vi "Combination Test.vi"() -> ()   [LabVIEW 2024]
uses:
  Log Record.ctl
  Logger/Internal Log Levels.ctl
  Filters/Match Behavior.ctl
  Filters/Aggregation Method.ctl
  5a9499bb-b307-4a4d-bae3-2140953a7cf6.vi
  5a9499bb-b307-4a4d-bae3-2140953a7cf6.vi/a153a250-4fb8-4a99-bb5b-6ccb57f1f631.vi
  5a9499bb-b307-4a4d-bae3-2140953a7cf6.vi/a153a250-4fb8-4a99-bb5b-6ccb57f1f631.vi/28727e37-b0d9-407c-a479-ab0b7779cd69.vi
  Filters/Regex/Regex.lvclass
  Handlers/File Handler/File Handler.lvclass
  Filters/Combination/Combination.lvclass
  Filters/Regex/New (Element).vi
  Registry/Log.vi
  Registry/Registry.lvlib
  Logger/Logger.lvclass
  Logging.lvlib
  Filters/Scopes/Scope/Scope.lvclass
panel:
  out "error out":errorcluster
  out "failures":T3(array[cluster]) {"Log Record"."timestamp" format="%<%x %.3X>T"}
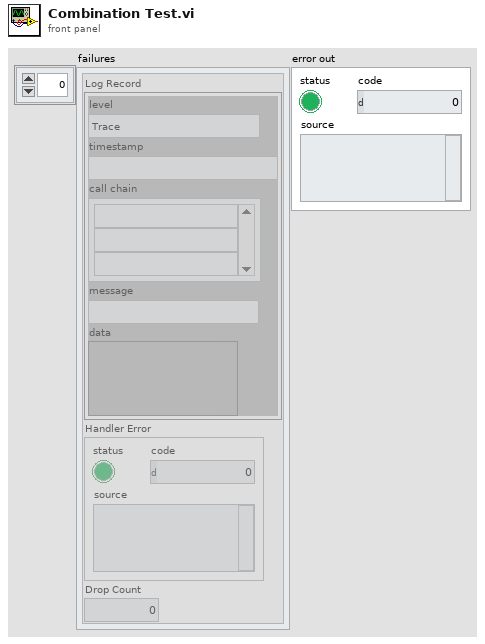
[diagram p1: front panel]
types:
  T1 = typedef "Logging.lvlib/Log Record.ctl" = cluster{"level":T2, "timestamp":timestamp, "call chain":string[], "message":string, "data":variant}
  T2 = typedef "Logging.lvlib/Internal Log Levels.ctl" = enum16{"Trace", "Debug", "Info", "Warning", "Error", "Critical", "Internal"}
  T3 = cluster{"Log Record":T1, "Handler Error":errorcluster, "Drop Count":u32}[]
  T4 = typedef "Logging.lvlib/Aggregation Method.ctl" = enum16{"Any", "Only", "All", "None"}
  T5 = typedef "Logging.lvlib/Match Behavior.ctl" = enum16{"Keep", "Discard"}
  T6 = cluster{"Log Record":T1, "Handler Error":errorcluster, "Drop Count":u32}
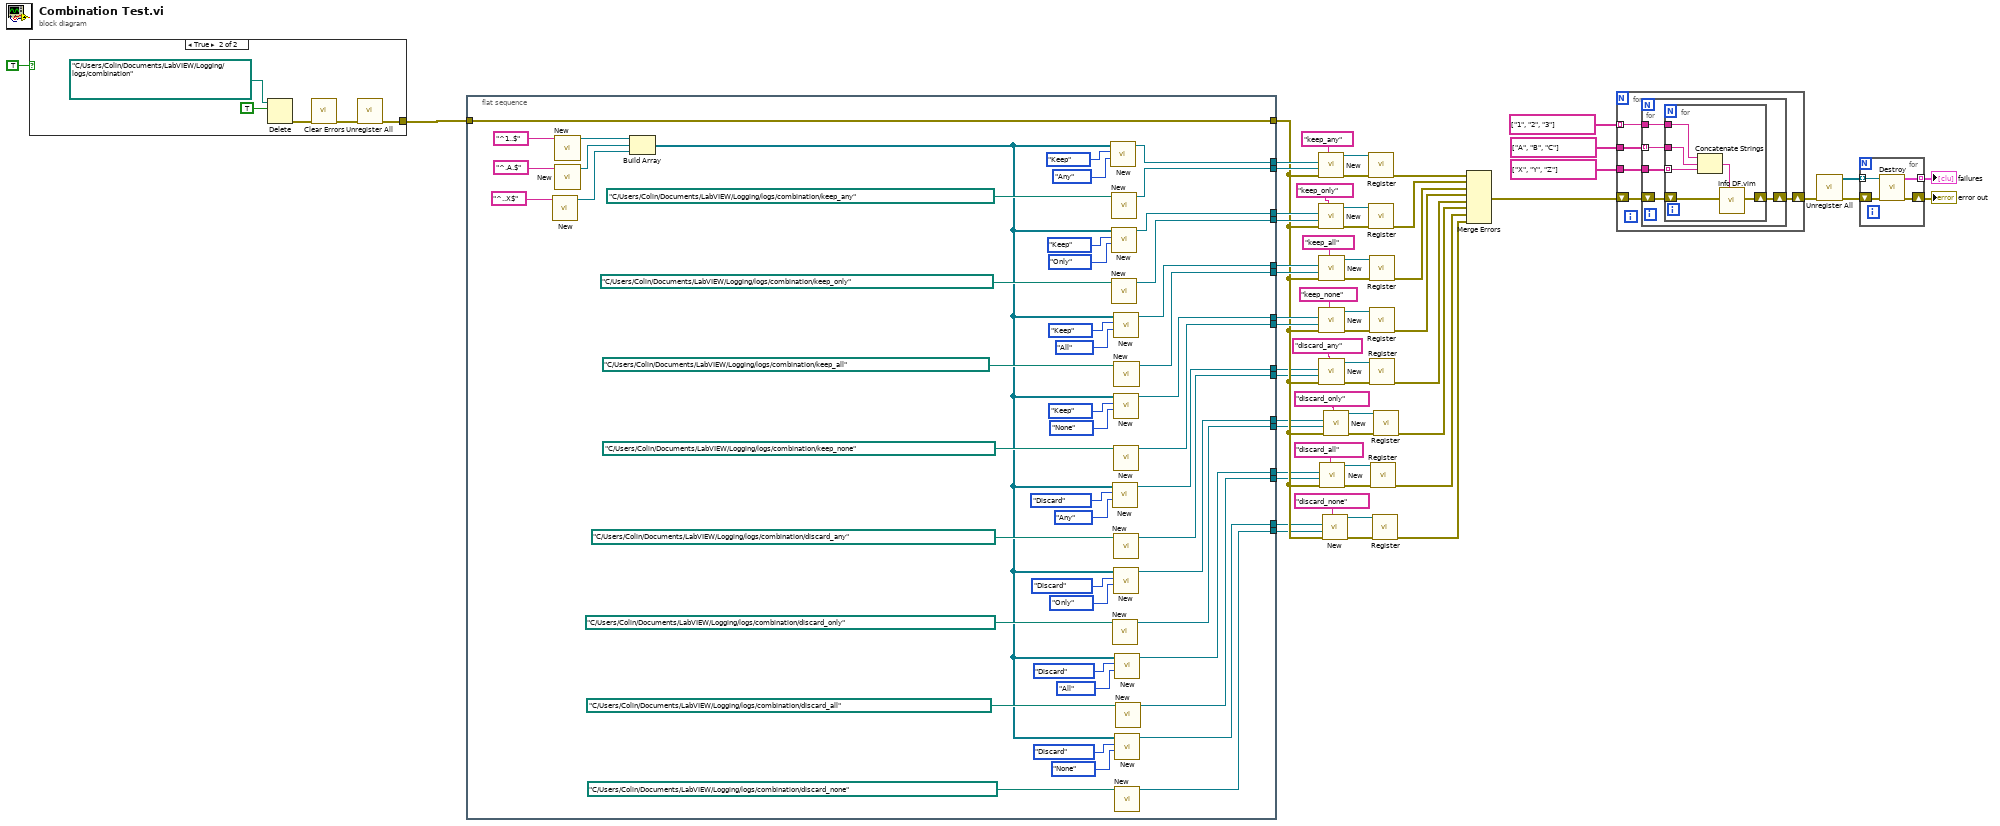
[diagram p0: block diagram]
diagram:
  n1 = case shown="True" TRUE {
    tunnel: [_ w61] -> w52
    frame False {
    }
    frame True {
      n2 = Delete(path (use dialog)=path "C:/Users/Colin/Documents/LabVIEW/Logging/logs/combination" ("log directory (<app dir>/logs)"), entire hierarchy (F)=TRUE) -> (error out=w64:errorcluster)  [unwired: 3 in, 2 out]
      n3 = call <vilib>:"Clear Errors.vi"("error in (no error)"=w64) -> ("error out"=w62:errorcluster)  [unwired: 5 in, 1 out]
      n4 = call "Unregister All.vi"("error in (no error)"=w62) -> ("error out"=w61:errorcluster)  [unwired: 9 in, 1 out]
    }
  }
  n5 = flat-sequence {
    tunnel: [w112] -> w60
    tunnel: w52 -> [w109]
    tunnel: [w109] -> w16
    tunnel: [w80] -> w44
    tunnel: [w79] -> w34
    tunnel: [w78] -> w33
    tunnel: [w77] -> w32
    tunnel: [w76] -> w31
    tunnel: [w75] -> w30
    tunnel: [w74] -> w29
    tunnel: [w73] -> w15
    tunnel: [w72] -> w14
    tunnel: [w71] -> w13
    tunnel: [w70] -> w12
    tunnel: [w69] -> w11
    tunnel: [w68] -> w10
    tunnel: [w67] -> w9
    tunnel: [w66] -> w8
    frame #0 {
      n6 = call-poly "New.vi"("regex string"="^..X$") -> ("regex out"=w105:refnum<class "Regex.lvclass">)  [unwired: 9 in, 1 out]
      n7 = call-poly "New.vi"("regex string"="^1..$") -> ("regex out"=w107:refnum<class "Regex.lvclass">)  [unwired: 9 in, 1 out]
      n8 = call-poly "New.vi"("regex string"="^.A.$") -> ("regex out"=w106:refnum<class "Regex.lvclass">)  [unwired: 9 in, 1 out]
      n9 = Build Array(w107, w106, w105) -> (w81:refnum<class "Regex.lvclass">[])
      n10 = call "New.vi"("aggregation method (any)"=Aggregation_Method."Any", "match behavior (keep)"=Match_Behavior."Keep", "sub-filters"=w81) -> ("aggregate filter"=w80:refnum<class "Combination.lvclass">)  [unwired: 8 in]
      n11 = call "New.vi"("log directory (<app dir>/logs)"=path "C:/Users/Colin/Documents/LabVIEW/Logging/logs/combination/keep_any") -> ("file handler"=w112:refnum<class "File Handler.lvclass">)  [unwired: 10 in]
      n12 = call "New.vi"("aggregation method (any)"=Aggregation_Method."Only", "match behavior (keep)"=Match_Behavior."Keep", "sub-filters"=w81) -> ("aggregate filter"=w79:refnum<class "Combination.lvclass">)  [unwired: 8 in]
      n13 = call "New.vi"("log directory (<app dir>/logs)"=path "C:/Users/Colin/Documents/LabVIEW/Logging/logs/combination/keep_only") -> ("file handler"=w78:refnum<class "File Handler.lvclass">)  [unwired: 10 in]
      n14 = call "New.vi"("aggregation method (any)"=Aggregation_Method."Any", "match behavior (keep)"=Match_Behavior."Discard", "sub-filters"=w81) -> ("aggregate filter"=w73:refnum<class "Combination.lvclass">)  [unwired: 8 in]
      n15 = call "New.vi"("log directory (<app dir>/logs)"=path "C:/Users/Colin/Documents/LabVIEW/Logging/logs/combination/discard_only") -> ("file handler"=w70:refnum<class "File Handler.lvclass">)  [unwired: 10 in]
      n16 = call "New.vi"("aggregation method (any)"=Aggregation_Method."All", "match behavior (keep)"=Match_Behavior."Keep", "sub-filters"=w81) -> ("aggregate filter"=w77:refnum<class "Combination.lvclass">)  [unwired: 8 in]
      n17 = call "New.vi"("aggregation method (any)"=Aggregation_Method."None", "match behavior (keep)"=Match_Behavior."Keep", "sub-filters"=w81) -> ("aggregate filter"=w75:refnum<class "Combination.lvclass">)  [unwired: 8 in]
      n18 = call "New.vi"("log directory (<app dir>/logs)"=path "C:/Users/Colin/Documents/LabVIEW/Logging/logs/combination/keep_none") -> ("file handler"=w74:refnum<class "File Handler.lvclass">)  [unwired: 10 in]
      n19 = call "New.vi"("log directory (<app dir>/logs)"=path "C:/Users/Colin/Documents/LabVIEW/Logging/logs/combination/discard_any") -> ("file handler"=w72:refnum<class "File Handler.lvclass">)  [unwired: 10 in]
      n20 = call "New.vi"("aggregation method (any)"=Aggregation_Method."Only", "match behavior (keep)"=Match_Behavior."Discard", "sub-filters"=w81) -> ("aggregate filter"=w71:refnum<class "Combination.lvclass">)  [unwired: 8 in]
      n21 = call "New.vi"("log directory (<app dir>/logs)"=path "C:/Users/Colin/Documents/LabVIEW/Logging/logs/combination/keep_all") -> ("file handler"=w76:refnum<class "File Handler.lvclass">)  [unwired: 10 in]
      n22 = call "New.vi"("aggregation method (any)"=Aggregation_Method."All", "match behavior (keep)"=Match_Behavior."Discard", "sub-filters"=w81) -> ("aggregate filter"=w69:refnum<class "Combination.lvclass">)  [unwired: 8 in]
      n23 = call "New.vi"("aggregation method (any)"=Aggregation_Method."None", "match behavior (keep)"=Match_Behavior."Discard", "sub-filters"=w81) -> ("aggregate filter"=w67:refnum<class "Combination.lvclass">)  [unwired: 8 in]
      n24 = call "New.vi"("log directory (<app dir>/logs)"=path "C:/Users/Colin/Documents/LabVIEW/Logging/logs/combination/discard_none") -> ("file handler"=w66:refnum<class "File Handler.lvclass">)  [unwired: 10 in]
      n25 = call "New.vi"("log directory (<app dir>/logs)"=path "C:/Users/Colin/Documents/LabVIEW/Logging/logs/combination/discard_all") -> ("file handler"=w68:refnum<class "File Handler.lvclass">)  [unwired: 10 in]
    }
  }
  n26 = call "New.vi"("name (\"Default\")"="keep_any" ("name (\"Default\")"), "error in (no error)"=w16, "log handler (file handler)"=w60, "log filter (none)"=w44) -> ("error out"=w58:errorcluster, "logger"=w59:refnum<class "Logger.lvclass">)  [unwired: 6 in]
  n27 = call "New.vi"("name (\"Default\")"="keep_only" ("name (\"Default\")"), "error in (no error)"=w16, "log handler (file handler)"=w33, "log filter (none)"=w34) -> ("error out"=w42:errorcluster, "logger"=w43:refnum<class "Logger.lvclass">)  [unwired: 6 in]
  n28 = call "New.vi"("name (\"Default\")"="keep_all" ("name (\"Default\")"), "error in (no error)"=w16, "log handler (file handler)"=w31, "log filter (none)"=w32) -> ("error out"=w39:errorcluster, "logger"=w38:refnum<class "Logger.lvclass">)  [unwired: 6 in]
  n29 = call "New.vi"("name (\"Default\")"="keep_none" ("name (\"Default\")"), "error in (no error)"=w16, "log handler (file handler)"=w29, "log filter (none)"=w30) -> ("error out"=w36:errorcluster, "logger"=w37:refnum<class "Logger.lvclass">)  [unwired: 6 in]
  n30 = call "New.vi"("name (\"Default\")"="discard_any" ("name (\"Default\")"), "error in (no error)"=w16, "log handler (file handler)"=w14, "log filter (none)"=w15) -> ("error out"=w27:errorcluster, "logger"=w28:refnum<class "Logger.lvclass">)  [unwired: 6 in]
  n31 = call "New.vi"("name (\"Default\")"="discard_all" ("name (\"Default\")"), "error in (no error)"=w16, "log handler (file handler)"=w10, "log filter (none)"=w11) -> ("error out"=w21:errorcluster, "logger"=w20:refnum<class "Logger.lvclass">)  [unwired: 6 in]
  n32 = call "New.vi"("name (\"Default\")"="discard_none" ("name (\"Default\")"), "error in (no error)"=w16, "log handler (file handler)"=w8, "log filter (none)"=w9) -> ("error out"=w18:errorcluster, "logger"=w19:refnum<class "Logger.lvclass">)  [unwired: 6 in]
  n33 = call "New.vi"("name (\"Default\")"="discard_only" ("name (\"Default\")"), "error in (no error)"=w16, "log handler (file handler)"=w12, "log filter (none)"=w13) -> ("error out"=w24:errorcluster, "logger"=w25:refnum<class "Logger.lvclass">)  [unwired: 6 in]
  n34 = call "Register.vi"("error in (no error)"=w58, "logger in"=w59) -> ("error out"=w56:errorcluster)  [unwired: 9 in]
  n35 = call "Register.vi"("error in (no error)"=w42, "logger in"=w43) -> ("error out"=w7:errorcluster)  [unwired: 9 in]
  n36 = call "Register.vi"("error in (no error)"=w39, "logger in"=w38) -> ("error out"=w6:errorcluster)  [unwired: 9 in]
  n37 = call "Register.vi"("error in (no error)"=w36, "logger in"=w37) -> ("error out"=w5:errorcluster)  [unwired: 9 in]
  n38 = call "Register.vi"("error in (no error)"=w27, "logger in"=w28) -> ("error out"=w4:errorcluster)  [unwired: 9 in]
  n39 = call "Register.vi"("error in (no error)"=w21, "logger in"=w20) -> ("error out"=w2:errorcluster)  [unwired: 9 in]
  n40 = call "Register.vi"("error in (no error)"=w18, "logger in"=w19) -> ("error out"=w1:errorcluster)  [unwired: 9 in]
  n41 = call "Register.vi"("error in (no error)"=w24, "logger in"=w25) -> ("error out"=w3:errorcluster)  [unwired: 9 in]
  n42 = Merge Errors(w56, w7, w6, w5, w4, w3, w2, w1) -> (w55:errorcluster)
  n43 = for {
    shift-right: [w117] -> w54
    shift-left: w55 -> [w118]
    tunnel: string[] ["1", "2", "3"] -> [w116] mode=indexing
    tunnel: string[] ["A", "B", "C"] -> [w115]
    tunnel: string[] ["X", "Y", "Z"] -> [w114]
    n44 = for {
      shift-right: [w122] -> w117
      shift-left: w118 -> [w123]
      tunnel: w116 -> [w121]
      tunnel: w115 -> [w120] mode=indexing
      tunnel: w114 -> [w119]
      n45 = for {
        shift-right: [w128] -> w122
        shift-left: w123 -> [w129]
        tunnel: w121 -> [w127]
        tunnel: w120 -> [w126]
        tunnel: w119 -> [w125] mode=indexing
        n46 = Concatenate Strings(w127, w126, w125) -> (w124:string)
        n47 = call "Info DF.vim"("message"=w124, "dataflow in"=w129) -> ("dataflow out"=w128:errorcluster)  [unwired: 9 in]
      }
    }
  }
  n48 = call "Unregister All.vi"("error in (no error)"=w54) -> ("error out"=w51:errorcluster, "loggers"=w50:refnum<class "Logger.lvclass">[])  [unwired: 9 in]
  n49 = for {
    tunnel: w50 -> [w132] mode=indexing
    tunnel: [w131] -> w49 mode=indexing
    shift-right: [w130] -> w48
    shift-left: w51 -> [w133]
    n50 = call "Destroy.vi"("error in (no error)"=w133, "logger in"=w132) -> ("error out"=w130:errorcluster, "fail info"=w131:T6)  [unwired: 8 in]
  }
  "failures" <- w49
  "error out" <- w48
